vi "hse-configuration_GetAllSections.vi"(8 "error in (no error)":errorcluster, 11 "hse-config-ini in":refnum<class "hse-config-ini.lvclass">) -> (0 "error out":errorcluster, 2 "Sections":string[](array[string]), 3 "hse-config-ini out":refnum<class "hse-config-ini.lvclass">)   [LabVIEW 2014, in "hse-config-ini.lvclass"]
doc: "Reads the numeric configuration value (DOUBLE) identified by <b>section</b> and <b>key</b> from the configuration object\n\n____\nHAMPEL SOFTWARE ENGINEERING v0.12.0 (2018-09-13 18:21)"
uses:
  hse-config-ini.lvclass
  hse-configuration.lvclass/hse-configuration.ctl
  hse-configuration_ReadDataDirectory.vi
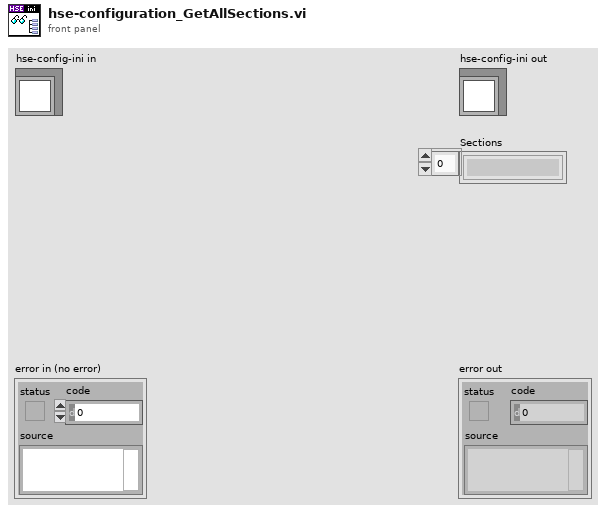
[diagram p1: front panel]
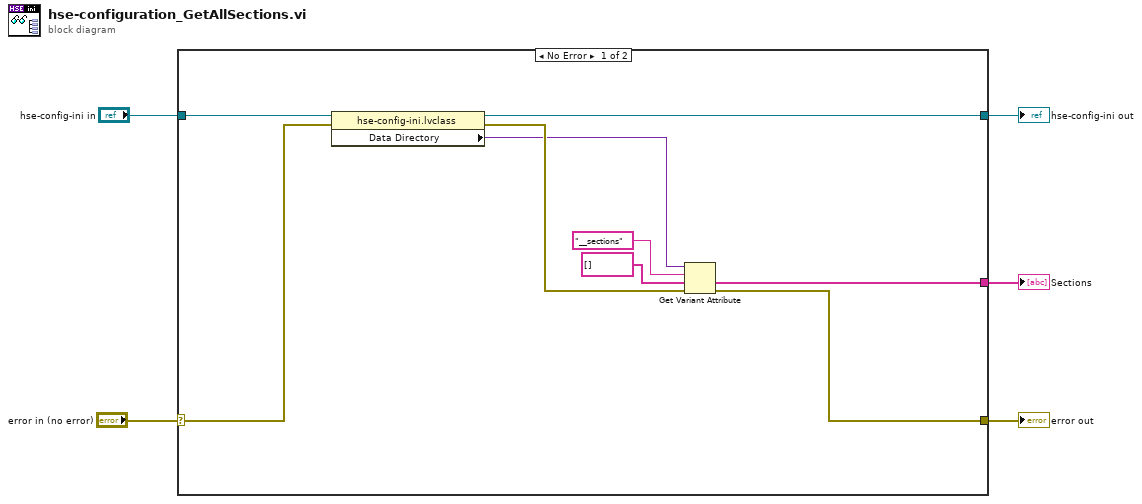
[diagram p0: block diagram]
diagram:
  n1 = case shown="No Error" "error in (no error)" {
    selector: "error in (no error)" -> [w12 w16]
    tunnel: [w10 w16] -> w2
    tunnel: "hse-config-ini in" -> [w14 w15]
    tunnel: [w13 w15] -> w3
    tunnel: [w6 _] -> w1
    frame No Error {
      n2 = property class="hse-config-ini.lvclass"(reference=w14, error in=w12) -> (reference out=w13:refnum<class "hse-config-ini.lvclass">, error out=w11:errorcluster, "Data Directory"=w9:variant)
      n3 = Get Variant Attribute(Variant=w9, name="__sections", default value (empty Variant)=string[] [] ("Sections"), error in=w11) -> (value=w6:string[], error out=w10:errorcluster)  [unwired: 2 out]
    }
    frame Error {
    }
  }
  "error out" <- w2
  "hse-config-ini out" <- w3
  "Sections" <- w1
